vi "Close Session.vi"(8 "error in":errorcluster, 11 "SR3XXX HVPS in":refnum<class "SR3XXX HVPS.lvclass">) -> (0 "error out":errorcluster, 3 "SR3XXX HVPS out":refnum<class "SR3XXX HVPS.lvclass">)   [LabVIEW 2014, in "SR3XXX HVPS.lvclass"]
uses:
  SR3XXX HVPS.lvclass
  Base/Session HVPS.lvclass
  reusable/Session APIs/Serial/Serial Session.lvclass
  reusable/Session APIs/Serial/Typedefs/Session Handle.ctl
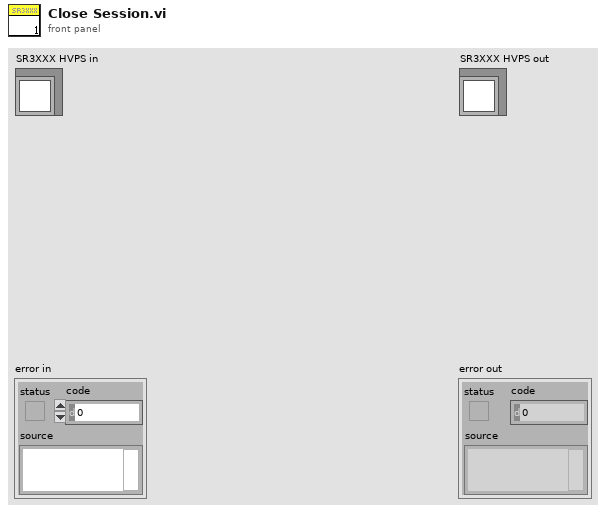
[diagram p1: front panel]
types:
  T1 = typedef "Serial Session.lvclass/Session Handle.ctl" = refnum<data-value>
  T2 = typedef "Session - Root.lvclass/Session Handle.ctl" = refnum<data-value>
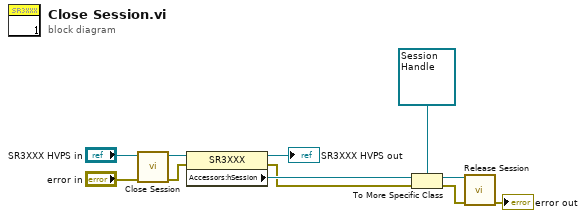
[diagram p0: block diagram]
diagram:
  n1 = call-parent "Close Session.vi"("error in"="error in", "Session HVPS in"="SR3XXX HVPS in") -> ("error out"=w8:errorcluster, "Session HVPS out"=w9:refnum<class "SR3XXX HVPS.lvclass">)  [unwired: 8 in]
  n2 = property class="SR3XXX"(reference=w9, error in=w8) -> (reference out=→"SR3XXX HVPS out":refnum<class "SR3XXX HVPS.lvclass">, error out=w5:errorcluster, "Accessors:hSession"=w6:T2)
  n3 = To More Specific Class(target class=T1 refnum ("Session Handle"), reference=w6, error in=w5) -> (specific class reference=w4:T1, error out=w3:errorcluster)
  n4 = call "Release Session.vi"("Session Handle"=w4, "error in (no error)"=w3) -> ("error out"=→"error out":errorcluster)  [unwired: 13 in]
